vi "run.vi"(8 "error in (no error)":errorcluster, 11 "Roda_Filtros in":refnum<class "Roda_Filtros.lvclass">) -> (0 "error out":errorcluster, 3 "Roda_Filtros out":refnum<class "Roda_Filtros.lvclass">)   [LabVIEW 2018, in "Roda_Filtros.lvclass"]
uses:
  Roda_Filtros.lvclass
  Roda_Filtros.lvclass/Roda_Filtros.ctl
  State Machine/State Machine.lvclass/State Machine.ctl
  State Machine/State Machine.lvclass
  RxTx/RxTx.lvclass
panel:
  out "Current Filter 2":u16(ring)=1 items=["Methane", "U", "B", "V", "R", "I", "Clear"]
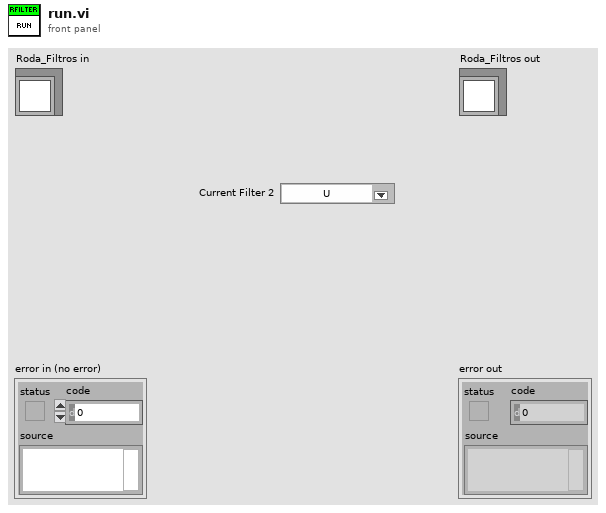
[diagram p1: front panel]
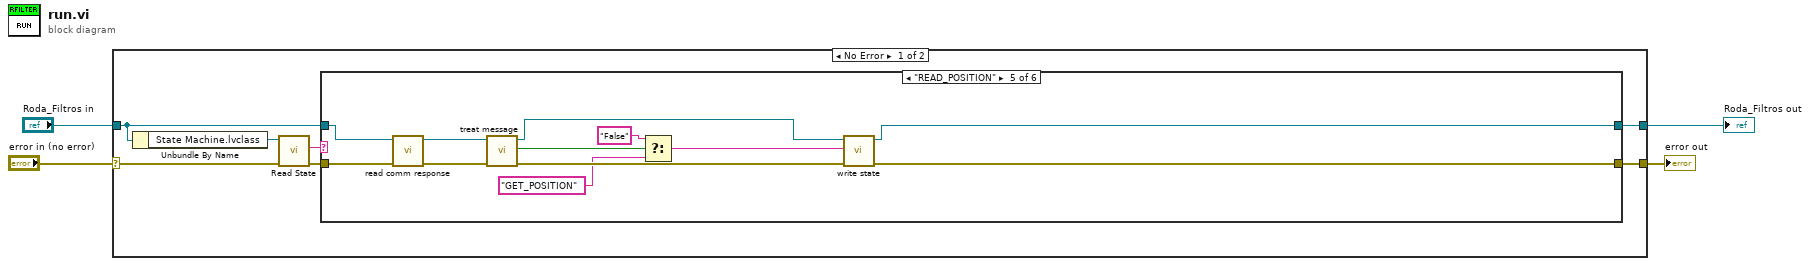
[diagram p0: block diagram]
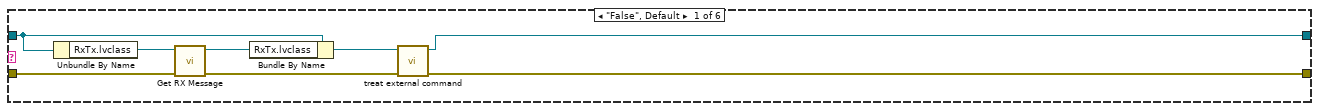
[diagram p2: hidden frame]
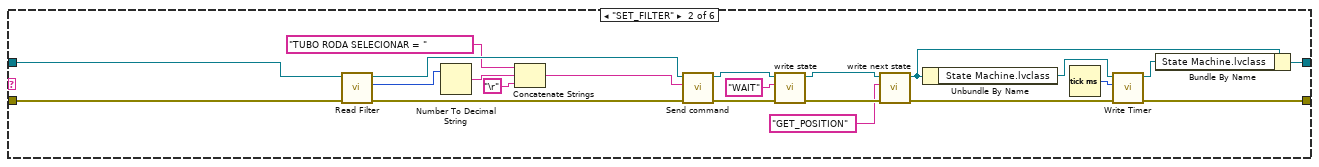
[diagram p3: hidden frame]
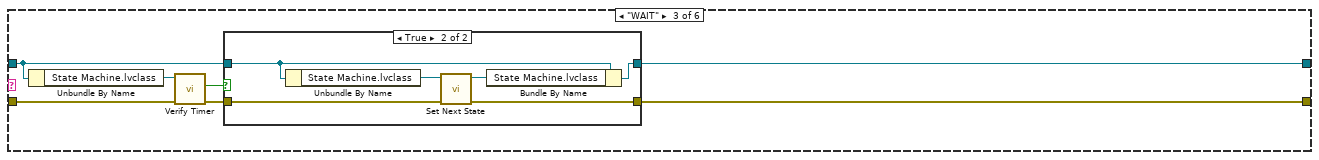
[diagram p4: hidden frame]
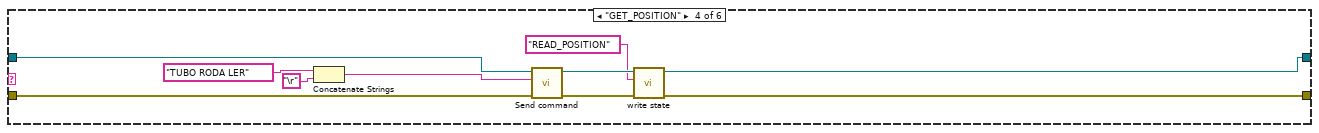
[diagram p6: hidden frame]
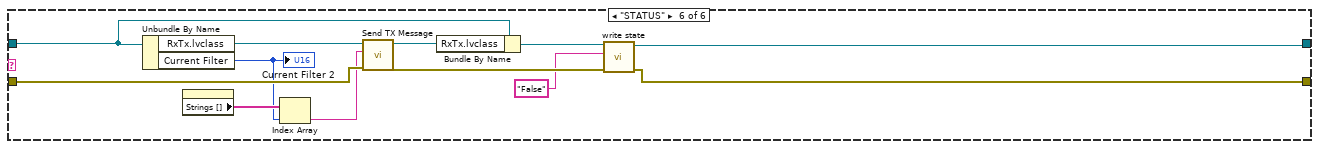
[diagram p7: hidden frame]
diagram:
  n1 = case shown="No Error" "error in (no error)" {
    selector: "error in (no error)" -> [w10 w92]
    tunnel: [w8 w92] -> w3
    tunnel: [w5 w91] -> w1
    tunnel: "Roda_Filtros in" -> [w6 w91]
    frame No Error {
      n2 = Unbundle By Name(w6) -> ("State Machine.lvclass"=w11:refnum<class "State Machine.lvclass">)
      n3 = call-dynamic "Read State.vi"("error in (no error)"=w10, "State Machine in"=w11) -> ("error out"=w9:errorcluster, "State"=w7:string)  [unwired: 7 in, 1 out]
      n4 = case shown="\"READ_POSITION\"" w7 {
        tunnel: [w12 w22 w43 w59 w75 w81] -> w8
        tunnel: w9 -> [w18 w40 w47 w65 w77 w89]
        tunnel: w6 -> [w16 w41 w45 w66 w78 w85]
        tunnel: [w13 w21 w42 w58 w76 w82] -> w5
        frame "False", Default {
          n5 = Unbundle By Name(w16) -> ("RxTx.lvclass"=w19:refnum<class "RxTx.lvclass">)
          n6 = call "Get RX Message.vi"("error in (no error)"=w18, "RxTx in"=w19) -> ("error out"=w15:errorcluster, "RxTx out"=w17:refnum<class "RxTx.lvclass">)  [unwired: 8 in]
          n7 = Bundle By Name(cluster=w16, "RxTx.lvclass"=w17) -> (w14:refnum<class "Roda_Filtros.lvclass">)
          n8 = call "treat external command.vi"("error in (no error)"=w15, "Roda_Filtros in"=w14) -> ("error out"=w12:errorcluster, "Roda_Filtros out"=w13:refnum<class "Roda_Filtros.lvclass">)  [unwired: 8 in]
        }
        frame "SET_FILTER" {
          n9 = call "Read Filter.vi"("error in (no error)"=w40, "Roda_Filtros in"=w41) -> ("error out"=w38:errorcluster, "Filter"=w35:u16, "Roda_Filtros out"=w39:refnum<class "Roda_Filtros.lvclass">)  [unwired: 7 in]
          n10 = Number To Decimal String(number=w35) -> (decimal integer string=w34:string)  [unwired: 1 in]
          n11 = Concatenate Strings("TUBO RODA SELECIONAR = " ("string"), w34, "\r") -> (w37:string)
          n12 = call "Send command.vi"("error in (no error)"=w38, "message"=w37, "Roda_Filtros in"=w39) -> ("error out"=w31:errorcluster, "Roda_Filtros out"=w32:refnum<class "Roda_Filtros.lvclass">)  [unwired: 7 in]
          n13 = call "write state.vi"("error in (no error)"=w31, "State"="WAIT", "Roda_Filtros in"=w32) -> ("error out"=w28:errorcluster, "Roda_Filtros out"=w29:refnum<class "Roda_Filtros.lvclass">)  [unwired: 7 in]
          n14 = call "write next state.vi"("error in (no error)"=w28, "Next State"="GET_POSITION" ("State"), "Roda_Filtros in"=w29) -> ("error out"=w23:errorcluster, "Roda_Filtros out"=w20:refnum<class "Roda_Filtros.lvclass">)  [unwired: 7 in]
          n15 = Unbundle By Name(w20) -> ("State Machine.lvclass"=w25:refnum<class "State Machine.lvclass">)
          n16 = Tick Count (ms)() -> (millisecond timer value=w24:u32)
          n17 = call "Write Timer.vi"("error in (no error)"=w23, "Timer"=w24, "State Machine in"=w25) -> ("error out"=w22:errorcluster, "State Machine out"=w26:refnum<class "State Machine.lvclass">)  [unwired: 7 in]
          n18 = Bundle By Name(cluster=w20, "State Machine.lvclass"=w26) -> (w21:refnum<class "Roda_Filtros.lvclass">)
        }
        frame "WAIT" {
          n19 = Unbundle By Name(w45) -> ("State Machine.lvclass"=w48:refnum<class "State Machine.lvclass">)
          n20 = call "Verify Timer.vi"("error in (no error)"=w47, "State Machine in"=w48) -> ("error out"=w44:errorcluster, "time out"=w46:bool)  [unwired: 7 in, 1 out]
          n21 = case shown="True" w46 {
            tunnel: w45 -> [w50 w56]
            tunnel: w44 -> [w49 w53]
            tunnel: [w49 w52] -> w43
            tunnel: [w50 w51] -> w42
            frame False {
            }
            frame True {
              n22 = Unbundle By Name(w56) -> ("State Machine.lvclass"=w54:refnum<class "State Machine.lvclass">)
              n23 = call "Set Next State.vi"("error in (no error)"=w53, "State Machine in"=w54) -> ("error out"=w52:errorcluster, "State Machine out"=w55:refnum<class "State Machine.lvclass">)  [unwired: 8 in]
              n24 = Bundle By Name(cluster=w56, "State Machine.lvclass"=w55) -> (w51:refnum<class "Roda_Filtros.lvclass">)
            }
          }
        }
        frame "GET_POSITION" {
          n25 = Concatenate Strings("TUBO RODA LER" ("string"), "\r") -> (w64:string)
          n26 = call "Send command.vi"("error in (no error)"=w65, "message"=w64, "Roda_Filtros in"=w66) -> ("error out"=w60:errorcluster, "Roda_Filtros out"=w61:refnum<class "Roda_Filtros.lvclass">)  [unwired: 7 in]
          n27 = call "write state.vi"("error in (no error)"=w60, "State"="READ_POSITION" ("string"), "Roda_Filtros in"=w61) -> ("error out"=w59:errorcluster, "Roda_Filtros out"=w58:refnum<class "Roda_Filtros.lvclass">)  [unwired: 7 in]
        }
        frame "READ_POSITION" {
          n28 = call "read comm response.vi"("error in (no error)"=w77, "Roda_Filtros in"=w78) -> ("error out"=w73:errorcluster, "Roda_Filtros out"=w74:refnum<class "Roda_Filtros.lvclass">)  [unwired: 8 in]
          n29 = call "treat message.vi"("error in (no error)"=w73, "Roda_Filtros in"=w74) -> ("error out"=w72:errorcluster, "filter positioned"=w68:bool, "Roda_Filtros out"=w71:refnum<class "Roda_Filtros.lvclass">)  [unwired: 7 in]
          n30 = Select(t="False" ("State"), s=w68, f="GET_POSITION" ("State")) -> (s? t:f=w69:string)
          n31 = call "write state.vi"("error in (no error)"=w72, "State"=w69, "Roda_Filtros in"=w71) -> ("error out"=w75:errorcluster, "Roda_Filtros out"=w76:refnum<class "Roda_Filtros.lvclass">)  [unwired: 7 in]
        }
        frame "STATUS" {
          n32 = Unbundle By Name(w85) -> ("RxTx.lvclass"=w90:refnum<class "RxTx.lvclass">, "Current Filter"=w87:u16)
          "Current Filter 2" <- w87
          n33 = property on="Current Filter 2" class="Ring (strict)"() -> ("Strings []"=w88:string[])  [unwired: 2 in, 2 out]
          n34 = Index Array(array=w88, index=w87) -> (element=w86:string)
          n35 = call "Send TX Message.vi"("error in (no error)"=w89, "element"=w86, "RxTx in"=w90) -> ("error out"=w80:errorcluster, "RxTx out"=w84:refnum<class "RxTx.lvclass">)  [unwired: 7 in]
          n36 = Bundle By Name(cluster=w85, "RxTx.lvclass"=w84) -> (w83:refnum<class "Roda_Filtros.lvclass">)
          n37 = call "write state.vi"("error in (no error)"=w80, "State"="False", "Roda_Filtros in"=w83) -> ("error out"=w81:errorcluster, "Roda_Filtros out"=w82:refnum<class "Roda_Filtros.lvclass">)  [unwired: 7 in]
        }
      }
    }
    frame Error {
    }
  }
  "error out" <- w3
  "Roda_Filtros out" <- w1
